vi "set x.vi"(10 "x":sgl, 11 "Vector 2D in":refnum<class "Vector 2D.lvclass">) -> (3 "Vector 2D out":refnum<class "Vector 2D.lvclass">)   [LabVIEW 2021, in "Vector 2D.lvclass"]
uses:
  Vector 2D.lvclass
  Vector 2D.lvclass/Vector 2D.ctl
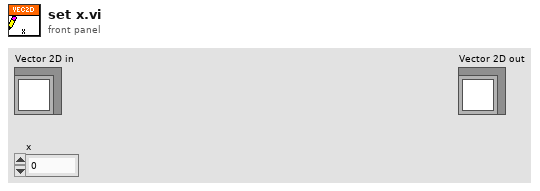
[diagram p1: front panel]
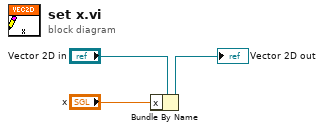
[diagram p0: block diagram]
diagram:
  n1 = Bundle By Name(cluster="Vector 2D in", "x"="x") -> (→"Vector 2D out":refnum<class "Vector 2D.lvclass">)
